vi "Write Alarm Limits.vi"(8 "error in":errorcluster, 10 "alarm limits":T1, 11 "Has Alarm Limits in":refnum<class "Has Alarm Limits.lvclass">) -> (0 "error out":errorcluster, 3 "Has Alarm Limits out":refnum<class "Has Alarm Limits.lvclass">)   [LabVIEW 2020, in "PV Access.lvlib" / "PV Data.lvlib" / "Has Alarm Limits.lvclass"]
uses:
  Has Alarm Limits.lvclass
  Alarm Severity.ctl
  PV Data.lvlib
  Alarm Limits.ctl
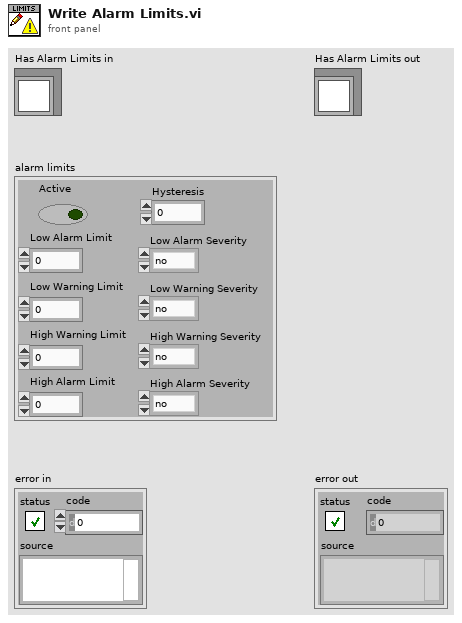
[diagram p1: front panel]
types:
  T1 = typedef "PV Access.lvlib/PV Data.lvlib/Alarm Limits.ctl" = cluster{"Active":bool, "Low Alarm Limit":dbl, "Low Warning Limit":dbl, "High Warning Limit":dbl, "High Alarm Limit":dbl, "Low Alarm Severity":T2, "Low Warning Severity":T2, "High Warning Severity ":T2, "High Alarm Severity":T2, "Hysteresis":dbl}
  T2 = typedef "PV Access.lvlib/PV Data.lvlib/Alarm Severity.ctl" = enum32{"no", "minor", "major", "record", "invalid", "undefined"}
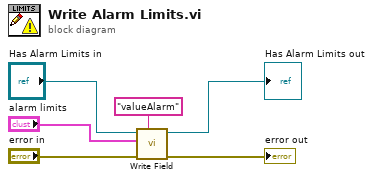
[diagram p0: block diagram]
diagram:
  n1 = call-dynamic "Write Field.vi"("field"="valueAlarm", "error in (no error)"="error in", "value"="alarm limits", "Base Interface in"="Has Alarm Limits in") -> ("error out"=→"error out":errorcluster, "Base Interface out"=→"Has Alarm Limits out":refnum<class "Has Alarm Limits.lvclass">)  [unwired: 6 in]
